vi "Update Focus.vi"(8 "error in (no error)":errorcluster, 10 "Focus region centers":dbl[](array[numeric]), 11 "Spectrum Recorder too in":refnum<class "Spectrum Recorder too.lvclass">) -> (0 "error out":errorcluster, 3 "Spectrum Recorder too out":refnum<class "Spectrum Recorder too.lvclass">)   [LabVIEW 2016, in "Spectrum Recorder too.lvclass"]
uses:
  Spectrum Recorder too.lvclass
  NHMFL_Core/Libraries/Red Pitaya/RP Core/Red Pitaya Transceiver Driver/Spectrum Configuration.ctl
  Write Spectrum Recorder Configuration.vi
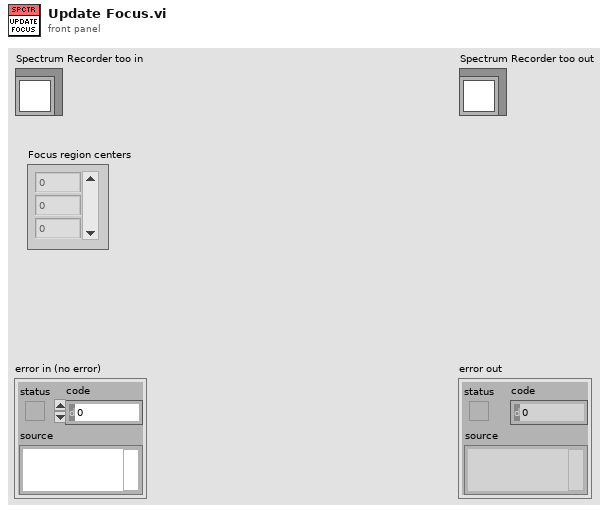
[diagram p1: front panel]
types:
  T1 = typedef "Spectrum Configuration.ctl" = cluster{"Start frequency":dbl, "End frequency":dbl, "Frequency step":dbl, "Step duration":dbl, "Red Pitaya address":string, "Open plot \non start":bool, "Focus region centers":dbl[], "Regions width":dbl, "Out-of-focus\nstep acceleration":i32}
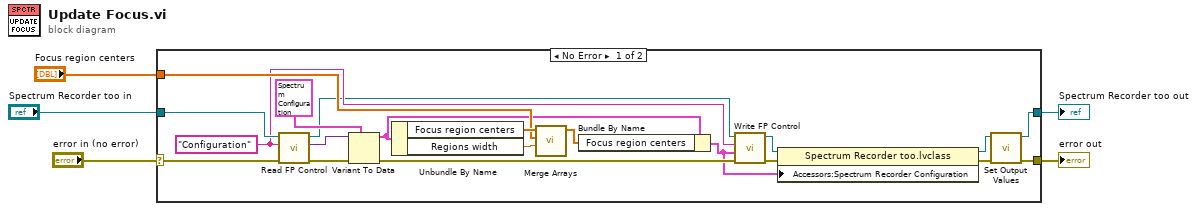
[diagram p0: block diagram]
diagram:
  n1 = case shown="No Error" "error in (no error)" {
    selector: "error in (no error)" -> [w13 w27]
    tunnel: [w10 w27] -> w4
    tunnel: [w12 w26] -> w2
    tunnel: "Spectrum Recorder too in" -> [w19 w26]
    tunnel: "Focus region centers" -> [w20 _]
    frame No Error {
      w16 = "Configuration" ("Control Name")
      n2 = call-dynamic "Read FP Control.vi"("error in (no error)"=w13, "Control Name"=w16, "Measure Object in"=w19) -> ("error out"=w25:errorcluster, "Control Value"=w24:variant, "Measure Object out"=w14:refnum<class "Spectrum Recorder too.lvclass">)  [unwired: 5 in, 1 out]
      n3 = Variant To Data(error in=w25, type=T1 {"Start frequency"=500000.0, "End frequency"=2000000.0, "Frequency step"=40.0, "Step duration"=0.004, "Red Pitaya address"="192.168.1.100", "Open plot \non start"=TRUE, "Focus region centers"=[], "Regions width"=2000.0, "Out-of-focus\nstep acceleration"=20} ("Configuration"), Variant=w24) -> (data=w18:T1, error out=w15:errorcluster)
      n4 = Unbundle By Name(w18) -> ("Focus region centers"=w22:dbl[], "Regions width"=w21:dbl)
      n5 = call "Merge Arrays.vi"("Coerce window width"=w21, "New Array"=w20, "Old Array"=w22) -> ("New Array out"=w17:dbl[])  [unwired: 8 in]
      n6 = Bundle By Name(cluster=w18, "Focus region centers"=w17) -> (w6:T1)
      n7 = call-dynamic "Write FP Control.vi"("error in (no error)"=w15, "Control Value"=w6, "Control Name"=w16, "Measure Object in"=w14) -> ("error out"=w11:errorcluster, "Measure Object out"=w8:refnum<class "Spectrum Recorder too.lvclass">)  [unwired: 6 in]
      n8 = property class="Spectrum Recorder too.lvclass"(reference=w8, error in=w11, "Accessors:Spectrum Recorder Configuration"=w6) -> (reference out=w7:refnum<class "Spectrum Recorder too.lvclass">, error out=w9:errorcluster)
      n9 = call-dynamic "Set Output Values.vi"("error in (no error)"=w9, "Spectrum Recorder in"=w7) -> ("error out"=w10:errorcluster, "Spectrum Recorder out"=w12:refnum<class "Spectrum Recorder too.lvclass">)  [unwired: 8 in]
    }
    frame Error {
    }
  }
  "error out" <- w4
  "Spectrum Recorder too out" <- w2
